vi "Frame Get w.vi"(8 "error in (no error)":errorcluster, 11 "IDE simple in":refnum<class "Main Panel.lvclass">) -> (0 "error out":errorcluster, 2 "<w> Data":T1, 3 "IDE simple out":refnum<class "Main Panel.lvclass">)   [LabVIEW 2018, in "Main Panel.lvlib" / "Main Panel.lvclass"]
uses:
  Main Panel.lvclass
  Frame Analizer/frame w data.ctl
  Main Panel.lvclass/Main Panel.ctl
  Frame Analizer/Data Parser.lvclass
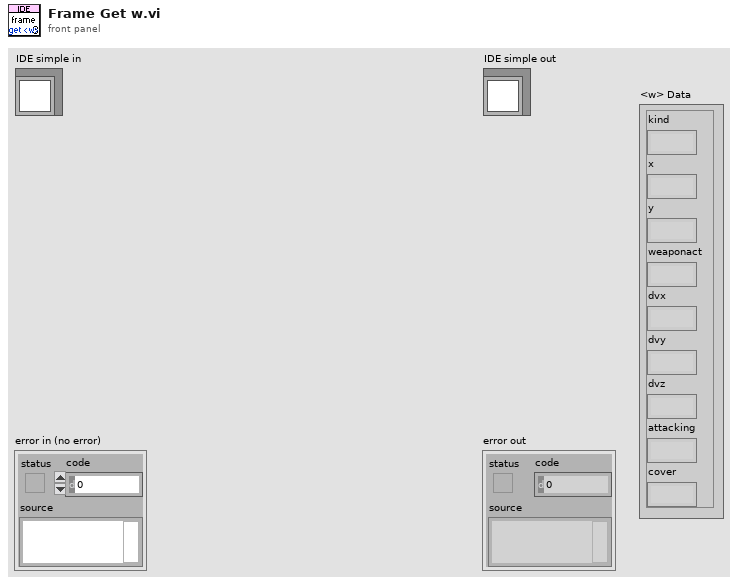
[diagram p1: front panel]
types:
  T1 = typedef "Data Parser.lvclass/frame w data.ctl" = cluster{"kind":string, "x":string, "y":string, "weaponact":string, "dvx":string, "dvy":string, "dvz":string, "attacking":string, "cover":string}
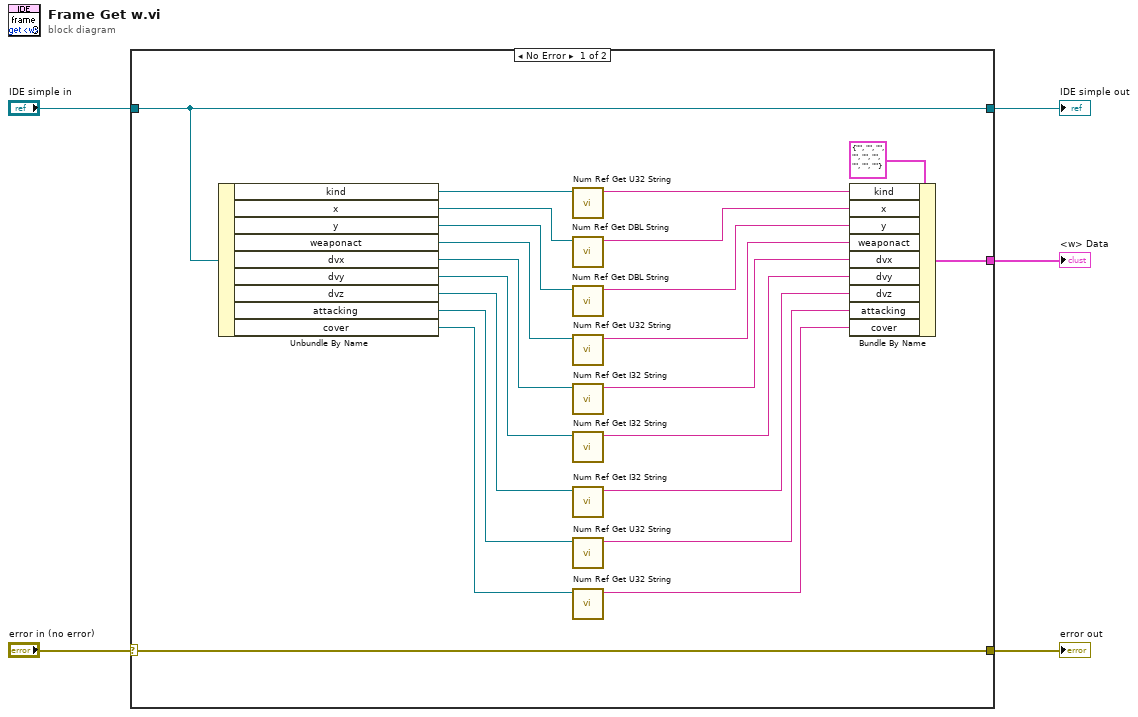
[diagram p0: block diagram]
diagram:
  n1 = case shown="No Error" "error in (no error)" {
    selector: "error in (no error)" -> [w15 w29]
    tunnel: [w15 w29] -> w4
    tunnel: [w27 w28] -> w2
    tunnel: "IDE simple in" -> [w27 w28]
    tunnel: [w26 _] -> w1
    frame No Error {
      n2 = Unbundle By Name(w27) -> ("kind"=w14:refnum<vi>, "x"=w13:refnum<vi>, "y"=w12:refnum<vi>, "weaponact"=w11:refnum<vi>, "dvx"=w10:refnum<vi>, "dvy"=w9:refnum<vi>, "dvz"=w8:refnum<vi>, "attacking"=w7:refnum<vi>, "cover"=w6:refnum<vi>)
      n3 = call "Num Ref Get U32 String.vi"("U32 Ref"=w14) -> ("Value string"=w24:string)  [unwired: 9 in, 1 out]
      n4 = call "Num Ref Get DBL String.vi"("DBL Ref"=w13) -> ("Value string"=w23:string)  [unwired: 9 in, 1 out]
      n5 = call "Num Ref Get DBL String.vi"("DBL Ref"=w12) -> ("Value string"=w22:string)  [unwired: 9 in, 1 out]
      n6 = call "Num Ref Get U32 String.vi"("U32 Ref"=w11) -> ("Value string"=w21:string)  [unwired: 9 in, 1 out]
      n7 = call "Num Ref Get I32 String.vi"("I32 Ref"=w10) -> ("Value String"=w20:string)  [unwired: 9 in, 1 out]
      n8 = call "Num Ref Get I32 String.vi"("I32 Ref"=w9) -> ("Value String"=w19:string)  [unwired: 9 in, 1 out]
      n9 = call "Num Ref Get I32 String.vi"("I32 Ref"=w8) -> ("Value String"=w18:string)  [unwired: 9 in, 1 out]
      n10 = call "Num Ref Get U32 String.vi"("U32 Ref"=w7) -> ("Value string"=w17:string)  [unwired: 9 in, 1 out]
      n11 = call "Num Ref Get U32 String.vi"("U32 Ref"=w6) -> ("Value string"=w16:string)  [unwired: 9 in, 1 out]
      n12 = Bundle By Name(cluster=T1 {"kind"="", "x"="", "y"="", "weaponact"="", "dvx"="", "dvy"="", "dvz"="", "attacking"="", "cover"=""} ("<w> data 2"), "kind"=w24, "x"=w23, "y"=w22, "weaponact"=w21, "dvx"=w20, "dvy"=w19, "dvz"=w18, "attacking"=w17, "cover"=w16) -> (w26:T1)
    }
    frame Error {
    }
  }
  "error out" <- w4
  "IDE simple out" <- w2
  "<w> Data" <- w1
